vi "GetAttributes.vi"(8 "error in (no error)":errorcluster, 11 "BrowerComposite in":refnum<class "BrowerComposite.lvclass">) -> (0 "error out":errorcluster, 2 "Attributes":variant, 3 "BrowerComposite out":refnum<class "BrowerComposite.lvclass">)   [LabVIEW 2015, in "BrowerComposite.lvclass"]
uses:
  BrowerComposite.lvclass
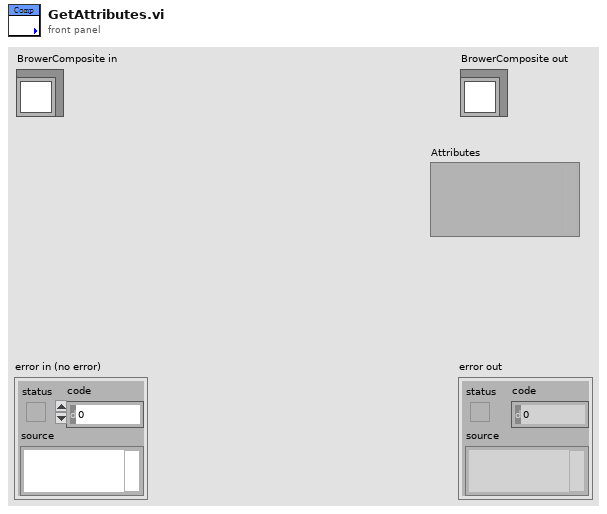
[diagram p1: front panel]
types:
  T1 = typedef "BrowerComposite.lvclass/ObjectAttributes.ctl" = cluster{"BrowerComponents":refnum<class "BrowerComponent.lvclass">[], "BrowerComponentIDs":string[], "Iterator":refnum<class "Iterator.lvclass">}
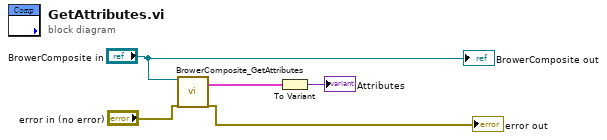
[diagram p0: block diagram]
diagram:
  n1 = call "BrowerComposite_GetAttributes.vi"("reference in"="BrowerComposite in", "error in (no error)"="error in (no error)") -> ("Data"=w2:T1, "error out"=→"error out":errorcluster)  [unwired: 14 in, 2 out]
  n2 = To Variant(anything=w2) -> (Variant=→"Attributes":variant)
  "BrowerComposite out" <- "BrowerComposite in"
